vi "NiFpga_HdlFifo32_AddI8.vi"(7 "direction":u32(ring)=1 items=["Target to Host", "Host to Target"], 8 "error in (no error)":errorcluster, 10 "Fifo Number":u32, 11 "FPGA VI Reference In":refnum<k20>) -> (0 "error out":errorcluster, 3 "FPGA VI Reference Out":refnum<k20>)   [LabVIEW 2023]
uses:
  NiFpga.dll
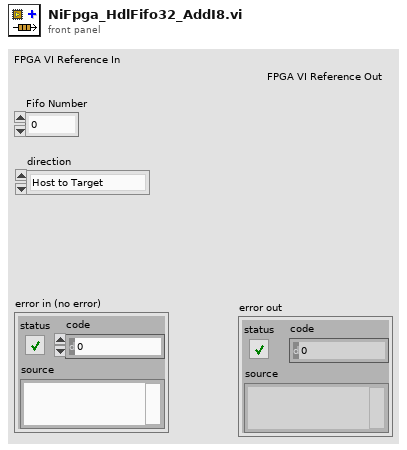
[diagram p1: front panel]
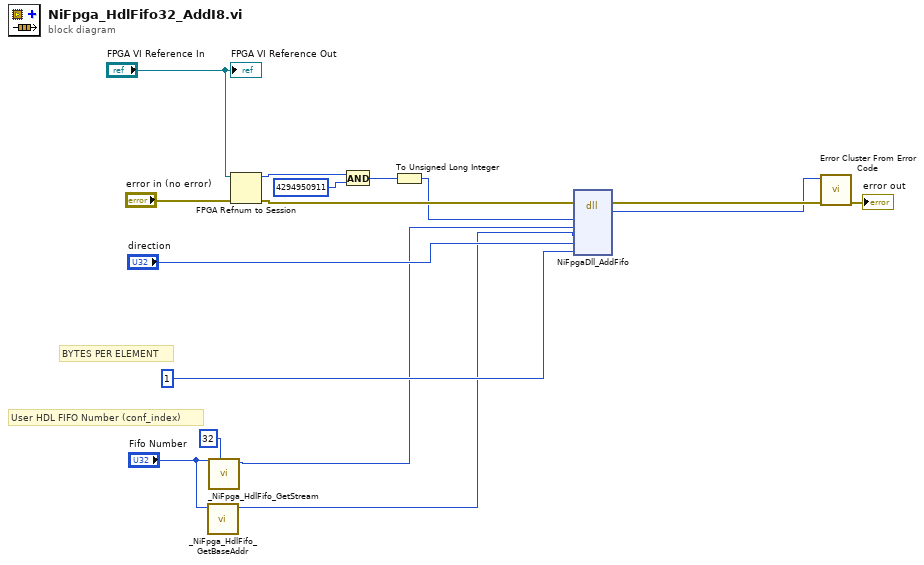
[diagram p0: block diagram]
diagram:
  # "BYTES PER ELEMENT"
  # "User HDL FIFO Number (conf_index)"
  n1 = call "_NiFpga_HdlFifo_GetBaseAddr.vi"("Fifo Number"="Fifo Number") -> ("Fifo Base Address"=w2:u32)  [unwired: 10 in]
  n2 = call "_NiFpga_HdlFifo_GetStream.vi"("NUM_DMA_CHANNELS"=u32 32, "Fifo Number"="Fifo Number") -> ("Fifo Stream"=w3:u32)  [unwired: 9 in]
  n3 = FPGA Refnum to Session(4:"error in (no error)", 7:"FPGA VI Reference In") -> (0:w11:errorcluster, 3:w13:u64)
  n4 = And(x=w13, y=u64 4294950911) -> (x .and. y?=w8:u64)
  n5 = To Unsigned Long Integer(number=w8) -> (unsigned 32bit integer=w7:u32)
  n6 = dll-call lib="NiFpga.*" fn="NiFpgaDll_AddFifo"(error in=w11, "session"=w7, "fifo"=w3, "baseAddress"=w2, "direction"="direction", "bytesPerElement"=u32 1) -> (error out=w10:errorcluster, "return type"=w9:i32)  [unwired: 7 in, 1 out]
  n7 = call <vilib>:"Error Cluster From Error Code.vi"("error in (no error)"=w10, "error code (0)"=w9) -> ("error out"=→"error out":errorcluster)  [unwired: 7 in]
  "FPGA VI Reference Out" <- "FPGA VI Reference In"
